vi "Coincident edges test.vi"(1 "epsilon":sgl, 2 "Edge 2":T1, 3 "Edge 1":T1) -> (0 "Edges are coincident":bool)   [LabVIEW 2014]
uses:
  Edge.ctl
panel:
  # "PN 21/03/2015"
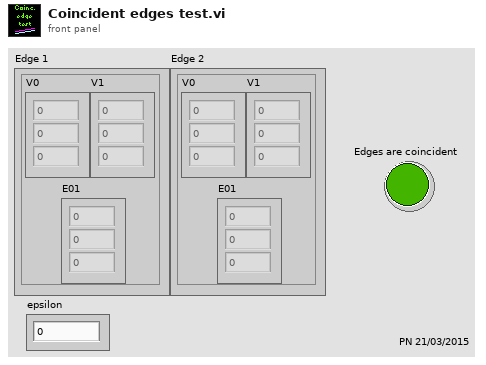
[diagram p1: front panel]
types:
  T1 = typedef "Edge.ctl" = cluster{"V0":sgl[], "V1":sgl[], "E01":sgl[]}
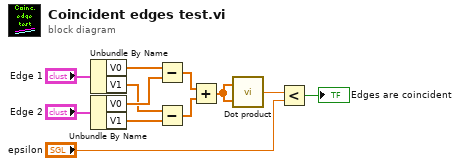
[diagram p0: block diagram]
diagram:
  n1 = Unbundle By Name("Edge 1") -> ("V0"=w10:sgl[], "V1"=w8:sgl[])
  n2 = Unbundle By Name("Edge 2") -> ("V0"=w9:sgl[], "V1"=w7:sgl[])
  n3 = Subtract(x=w10, y=w9) -> (x-y=w6:sgl[])
  n4 = Subtract(x=w8, y=w7) -> (x-y=w5:sgl[])
  n5 = Add(x=w6, y=w5) -> (x+y=w4:sgl[])
  n6 = call "Dot product.vi"("B"=w4, "A"=w4) -> ("A . B"=w3:sgl)
  n7 = Less?(x=w3, y="epsilon") -> (x < y?=→"Edges are coincident":bool)
